vi "CANOpen_Main_Write RPDOs.vi"(7 "Node states":u16[](array[ring]) items=["unknown"=1, "bootup"=0, "stopped"=4, "operational"=5, "pre-operational"=127, "connection lost"=128], 8 "error in (no error)":errorcluster, 9 "Data":dbl[](array[numeric]), 10 "Nodes":T4[](array[typedef]) {"NMT"."Node init static SDO state" items=["start remote node"=1, "enter pre-operational"=128]; "NMT"."Node run state" items=["start remote node"=1, "stop remote node"=2, "enter pre-operational"=128, "reset node"=129, "reset communication"=130]; "Dynamic SDOs"."Sub-Index (0)" format="%.0x"; "Dynamic SDOs"."Object Index" format="%.0x"; "Dynamic SDOs"."Block Data" format="%.0x"; "RPDOs"."PDO Channel" items=["PDO 1", "PDO 2", "PDO 3", "PDO 4"]; "RPDOs"."Parameters"."Bit Offset" max=8 step=1; "RPDOs"."Parameters"."Byte Offset" max=8 step=1; "TPDOs"."PDO Channel" items=["PDO 1", "PDO 2", "PDO 3", "PDO 4"]; "TPDOs"."Parameters"."Bit Offset" max=8 step=1; "TPDOs"."Parameters"."Byte Offset" max=8 step=1; "SDOs"."Sub-Index (0)" format="%.0x"; "SDOs"."Object Index" format="%.0x"; "SDOs"."Block Data" format="%.0x"}, 11 "xPDO Refs":T1) -> (0 "error out":errorcluster)   [LabVIEW 2021, in "CANOpen Addon Engine.lvlib"]
uses:
  CANOpen Addon Engine.lvlib
  SubVIS/CANOpen_Node Message Settings.ctl
  Shared/CANOpen_PDO Settings.ctl
  Shared/CANOpen_PDO Parameter Settings.ctl
  Shared/CANOpen_PDO Data Type.ctl
  System Explorer/SubVIs/CANopen Byte Order.ctl
  Shared/CANOpen_SDO Settings.ctl
  SubVIS/CANOpen_NMT Settings.ctl
  CanOpen_NMT_Config.ctl
  CanOpen_NMT_Static detect.ctl
  CANOpen_xPDO Refs.ctl
  CanOpen_RPDO Refs.ctl
  CanOpen_TPDO Refs.ctl
  Shared/CANOpen Addon Shared.lvlib
  System Explorer/CANOpen Addon System Explorer.lvlib
panel:
  # "LSB"
  # "MSB"
  # "LSB"
  # "MSB"
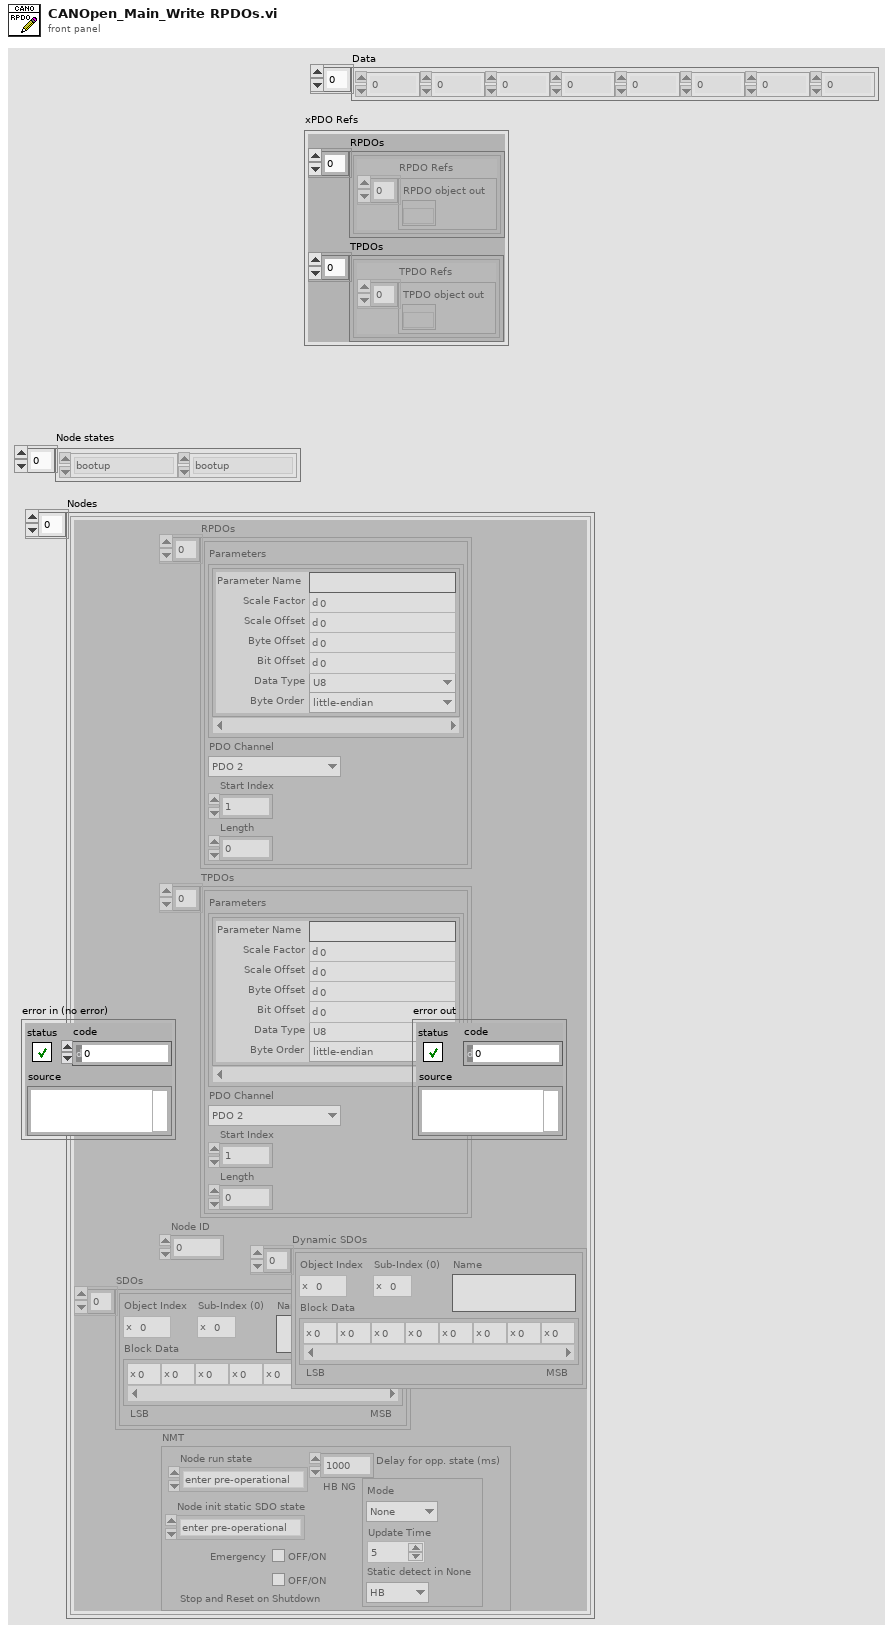
[diagram p1: front panel]
types:
  T1 = typedef "CANOpen Addon Engine.lvlib/CANOpen_xPDO Refs.ctl" = cluster{"RPDOs":T2[], "TPDOs":T3[]}
  T2 = typedef "CANOpen Addon Engine.lvlib/CanOpen_RPDO Refs.ctl" = cluster{"RPDO Refs":refnum<k20>[]}
  T3 = typedef "CANOpen Addon Engine.lvlib/CanOpen_TPDO Refs.ctl" = cluster{"TPDO Refs":refnum<k20>[]}
  T4 = typedef "CANOpen Addon Engine.lvlib/CANOpen_Node Message Settings.ctl" = cluster{"RPDOs":T5[], "TPDOs":T5[], "Node ID":u8, "SDOs":T9[], "Dynamic SDOs":T9[], "NMT":T10}
  T5 = typedef "CANOpen Addon Shared.lvlib/CANOpen_PDO Settings.ctl" = cluster{"Parameters":T6[], "PDO Channel":u8, "Start Index":u32, "Length":u32}
  T6 = typedef "CANOpen Addon Shared.lvlib/CANOpen_PDO Parameter Settings.ctl" = cluster{"Parameter Name":string, "Scale Factor":dbl, "Scale Offset":dbl, "Byte Offset":u8, "Bit Offset":u8, "Data Type":T7, "Byte Order":T8}
  T7 = typedef "CANOpen Addon Shared.lvlib/CANOpen_PDO Data Type.ctl" = enum16{"U8", "U16", "U32", "I8", "I16", "I32", "Single", "Double", "Boolean"}
  T8 = typedef "CANOpen Addon System Explorer.lvlib/CANopen Byte Order.ctl" = enum16{"big-endian network order", "little-endian"}
  T9 = typedef "CANOpen Addon Shared.lvlib/CANOpen_SDO Settings.ctl" = cluster{"Object Index":u16, "Sub-Index (0)":u8, "Block Data":u8[], "Name":string}
  T10 = typedef "CANOpen Addon Engine.lvlib/CANOpen_NMT Settings.ctl" = cluster{"Node run state":u16, "Emergency":bool, "HB NG":T11, "Delay for opp. state (ms)":dbl, "Node init static SDO state":u16, "Stop and Reset on Shutdown":bool}
  T11 = typedef "CANOpen Addon Engine.lvlib/CanOpen_NMT_Config.ctl" = cluster{"Mode":T12, "Update Time":u16, "Static detect in None":T12}
  T12 = typedef "CANOpen Addon Engine.lvlib/CanOpen_NMT_Static detect.ctl" = enum16{"None", "HB", "NG"}
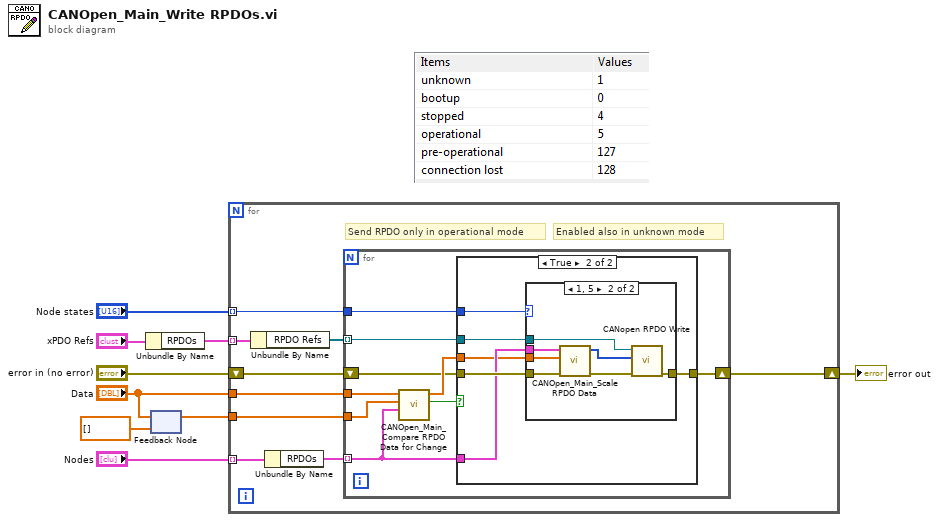
[diagram p0: block diagram]
diagram:
  n1 = Unbundle By Name("xPDO Refs") -> ("RPDOs"=w5:T2[])
  n2 = feedback-in #1("Data") -> ()
  n3 = feedback #1(dbl[] [] ("element out")) -> (w3:dbl[])
  n4 = for {
    tunnel: w5 -> [w15] mode=indexing
    tunnel: "Nodes" -> [w10] mode=indexing
    shift-right: [w18] -> w7
    shift-left: "error in (no error)" -> [w17]
    tunnel: "Data" -> [w13]
    tunnel: w3 -> [w12]
    tunnel: "Node states" -> [w11] mode=indexing
    # "Enabled also in unknown mode"
    # "Send RPDO only in operational mode"
    n5 = Unbundle By Name(w15) -> ("RPDO Refs"=w14:refnum<k20>[])
    n6 = Unbundle By Name(w10) -> ("RPDOs"=w16:T5[])
    n7 = for {
      tunnel: w14 -> [w27] mode=indexing
      shift-right: [w26] -> w18
      shift-left: w17 -> [w20]
      tunnel: w16 -> [w23] mode=indexing
      tunnel: w13 -> [w25]
      tunnel: w12 -> [w24]
      tunnel: w11 -> [w19]
      n8 = call "CANOpen_Main_Compare RPDO Data for Change.vi"("PDO Settings"=w23, "Previous Data"=w24, "Current Data"=w25) -> ("Changed?"=w22:bool, "Data"=w21:dbl[])  [unwired: 7 in]
      n9 = case shown="True" w22 {
        tunnel: w27 -> [_ w34]
        tunnel: [w28 w33] -> w26
        tunnel: w20 -> [w28 w32]
        tunnel: w23 -> [_ w31]
        tunnel: w21 -> [_ w30]
        tunnel: w19 -> [_ w29]
        frame False {
        }
        frame True {
          n10 = case shown="1, 5" w29 {
            tunnel: w34 -> [_ w42]
            tunnel: [w35 w41] -> w33
            tunnel: w32 -> [w35 w39]
            tunnel: w31 -> [_ w38]
            tunnel: w30 -> [_ w37]
            frame 0, Default {
            }
            frame 1, 5 {
              n11 = call "CANOpen_Main_Scale RPDO Data.vi"("error in (no error)"=w39, "Data"=w37, "PDO Settings"=w38) -> ("error out"=w36:errorcluster, "CANopen data out"=w40:u8[])  [unwired: 7 in]
              n12 = call <vilib>:"CANopen RPDO Write.vi"("error in (no error)"=w36, "data"=w40, "RPDO object in"=w42) -> ("error out"=w41:errorcluster)  [unwired: 7 in, 1 out]
            }
          }
        }
      }
    }
  }
  "error out" <- w7
